vi "RegExpTranslate.vi"(11 "string":string) -> (3 "regexp safe string":string)   [LabVIEW 2019, in "infolib.lvlib"]
doc: "Translate a string for use in regular expression."
uses:
  infolib.lvlib
panel:
  # "testing string:"
  # "haha\n.^$*+?()[{\\|\nhoho\n(Hz)"
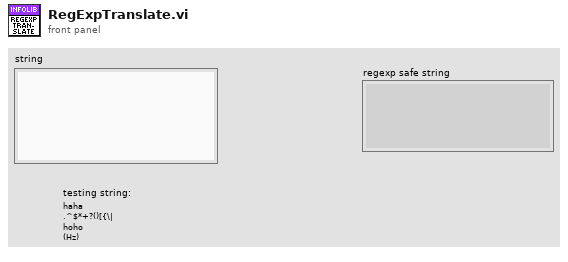
[diagram p1: front panel]
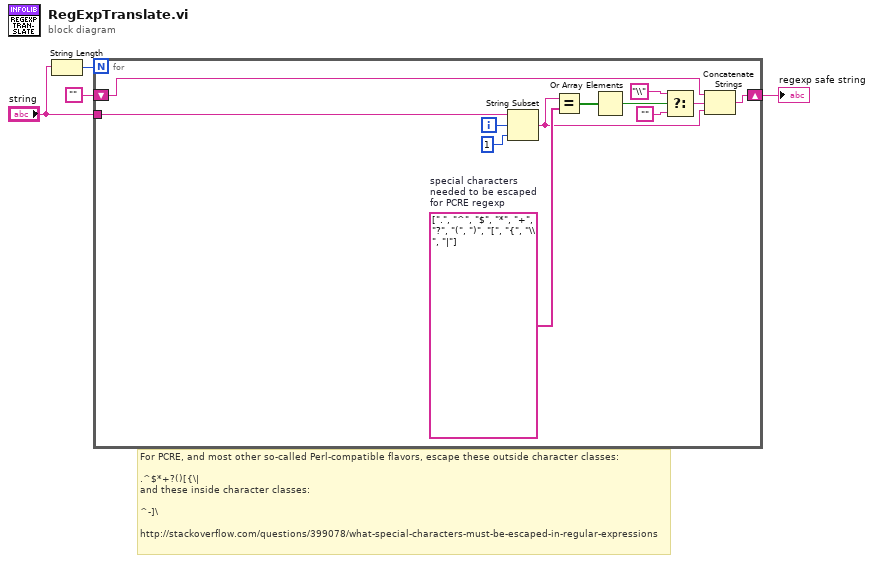
[diagram p0: block diagram]
diagram:
  # "For PCRE, and most other so-called Perl-compatible flavors, escape these outside character classes:\n\n.^$*+?()[{\\|\nand these inside character classes:\n\n^-]\\\n\nhttp://stackoverflow.com/questions/399078/what-special-characters-must-be-escaped-in-regular-expressions"
  n1 = String Length(string="string") -> (length=w3:i32)
  n2 = for {
    N: w3 -> [_]
    tunnel: "string" -> [w16]
    shift-right: [w6] -> w1
    shift-left: "" -> [w7]
    i -> [w15]
    w13 = string[] [".", "^", "$", "*", "+", "?", "(", ")", "[", "{", "\\", "|"]  # special characters needed to be escaped for PCRE regexp
    n3 = String Subset(string=w16, offset (0)=w15, length (rest)=1 ("length (rest)")) -> (substring=w5:string)
    n4 = Equal?(x=w5, y=w13) -> (x = y?=w12:bool[])
    n5 = Or Array Elements(Boolean array=w12) -> (logical OR=w11:bool)
    n6 = Select(t="\\" ("string"), s=w11, f="") -> (s? t:f=w8:string)
    n7 = Concatenate Strings(w7, w8, w5) -> (w6:string)
  }
  "regexp safe string" <- w1
